vi "Standby Power Search Replace 2D Array.vi"(8 "Error In":errorcluster, 9 "Insert Value":string="Linear Regression Stable", 10 "Search Element":string="Stop Factor", 11 "Array in in":string[][](array[string])) -> (0 "Error Out":errorcluster, 3 "Array out":string[][](array[string]))   [LabVIEW 2020]
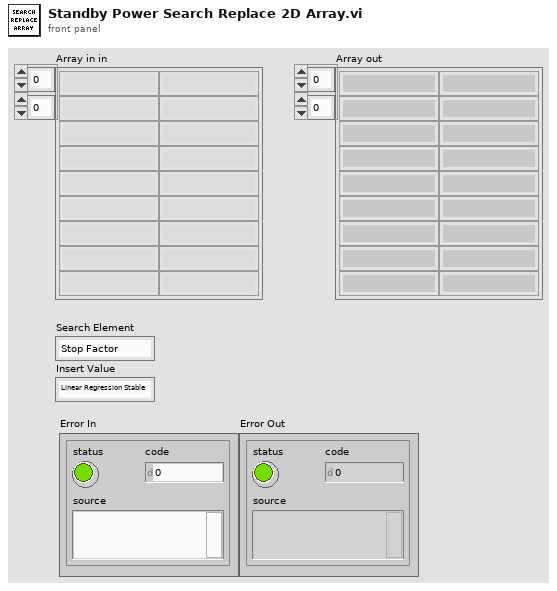
[diagram p1: front panel]
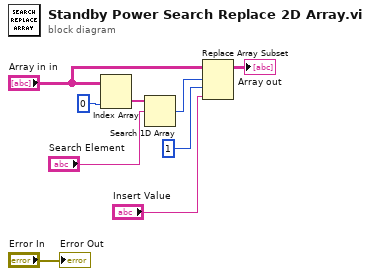
[diagram p0: block diagram]
diagram:
  n1 = Index Array(array="Array in in", index (col)=0 ("disabled index (col)")) -> (element=w5:string[])  [unwired: 1 in]
  n2 = Search 1D Array(1D array=w5, element="Search Element") -> (index of element=w8:i32)  [unwired: 1 in]
  n3 = Replace Array Subset(array="Array in in", new element="Insert Value", index (row)=w8, index (col)=1 ("disabled index (col)")) -> (→"Array out":string[][])
  "Error Out" <- "Error In"
